vi "fileManager.vi"() -> ()   [LabVIEW 2009]
panel:
  out "appended array":dbl[](array[numeric])=[9.99999e+37, 9.99999e+37, 2.137332e-09, 7.2166e-11, 9.99999e+37, 9.99999e+37, 9.99999e+37, 9.99999e+37, 9.99999e+37, 9.99999e+37, 15.0]
  out "String":string
  in  "Path":path
  out "error out":errorcluster
  in  "error in":errorcluster
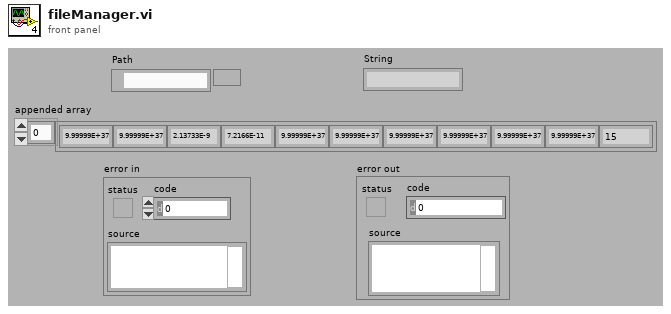
[diagram p1: front panel]
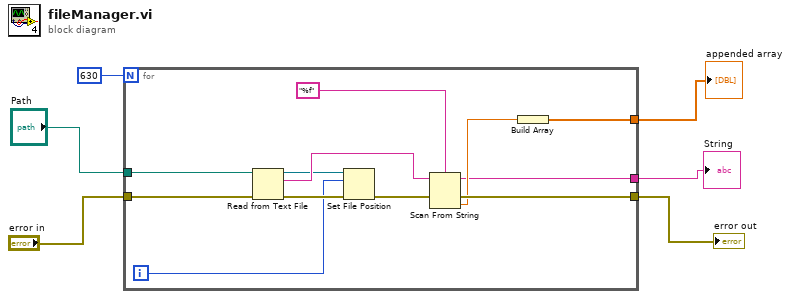
[diagram p0: block diagram]
diagram:
  n1 = for {
    N: 630 -> [_]
    tunnel: "error in" -> [w18]
    tunnel: [w13] -> w5
    tunnel: "Path" -> [w17]
    tunnel: [w14] -> w2
    tunnel: [w7] -> w1
    i -> [w8]
    n2 = Read from Text File(file (use dialog)=w17, error in=w18) -> (refnum out=w11:refnum<file>, text=w16:string, error out=w10:errorcluster)  [unwired: 2 in, 1 out]
    n3 = Set File Position(offset (in bytes) (0)=w8, refnum=w11, error in=w10) -> (error out=w9:errorcluster)  [unwired: 1 in, 1 out]
    n4 = Scan From String(format string="%f", input string=w16, error in=w9) -> (remaining string=w7:string, error out=w13:errorcluster, output 1=w12:dbl)  [unwired: 2 in, 1 out]
    n5 = Build Array(w12) -> (w14:dbl[])
  }
  "error out" <- w5
  "String" <- w1
  "appended array" <- w2
